vi "Simple H5Dwrite (Variant).vi"(0 "HDF5 Location Ref":T2, 1 "Close Dataset (T)":bool=TRUE, 2 "Compression Level (0-disabled)":i32 min=0 max=9 step=1, 3 "Chunk size":i32[](array[numeric]), 5 "Dataset Path":string, 9 "Unlimited  dataset (F)":bool, 11 "error in (no error)":errorcluster, 12 "operation (open or create)":T1=enum."open or create", 14 "Data":variant) -> (4 "HDF5 Location Ref out":T2, 6 "HDF5 Dataset Ref out":T2, 15 "error out":errorcluster)   [LabVIEW 2017]
doc: "Writes data into a dataset."
uses:
  <vilib>/UPVI/lvhdf5/library.llb/HDF5 Ref.ctl
  <vilib>/UPVI/lvhdf5/dataset.llb/LVH5D Operation.ctl
  <vilib>/UPVI/lvhdf5/common.llb/To HDF5 Ref.vi
panel:
  # "LVHDF5 Toolkit\nCopyright (c) 2005-2013 by Jason D. Sommerville\nCopyright (c) 2014 by UPVI, LLC.\n\nThis use and distribution of this file is governed by the terms found in \nLICENSE.txt distributed with this toolkit and installed at\n <user.lib>\\_lvhdf5\\LICENSE.txt"
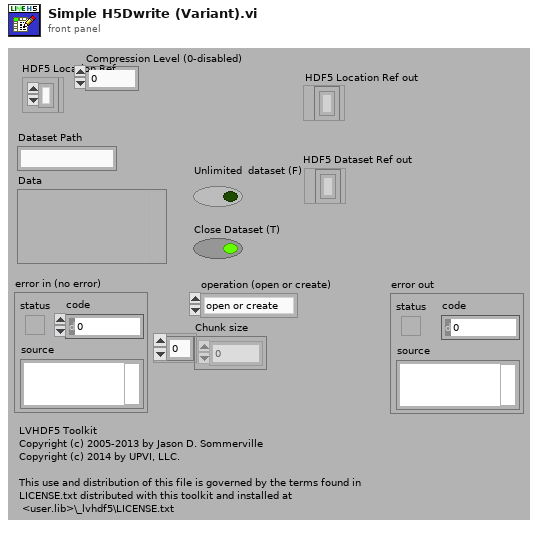
[diagram p1: front panel]
types:
  T1 = typedef "LVH5D Operation.ctl" = enum16{"open", "replace", "create", "open or create", "create or replace", "create or replace with confirmation"}
  T2 = typedef "HDF5 Ref.ctl" = refnum<k1>
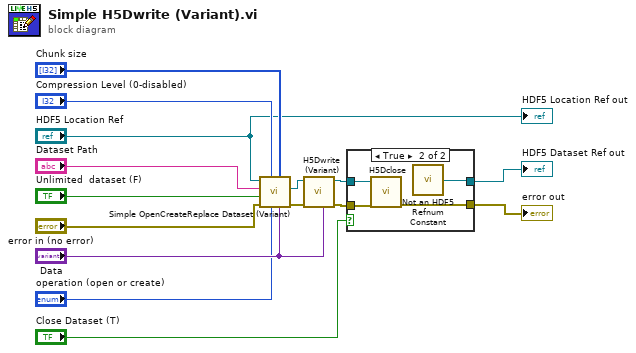
[diagram p0: block diagram]
diagram:
  n1 = call <vilib>:"Simple OpenCreateReplace Dataset (Variant).vi"("Datatype and Dataspace"="Data", "Chunk size"="Chunk size", "operation (open or create)"="operation (open or create)", "Compression Level (0-disabled)"="Compression Level (0-disabled)", "error in (no error)"="error in (no error)", "Unlimited  dataset (F)"="Unlimited  dataset (F)", "Dataset Path"="Dataset Path", "HDF5 Ref"="HDF5 Location Ref") -> ("error out"=w1:errorcluster, "HDF5 Dataset Ref out"=w2:T2)  [unwired: 1 in, 1 out]
  n2 = call <vilib>:"H5Dwrite (Variant).vi"("Data"="Data", "error in (no error)"=w1, "HDF5 Dataset Ref"=w2) -> ("error out"=w3:errorcluster, "HDF5 Ref out"=w4:T2)  [unwired: 7 in]
  n3 = case shown="True" "Close Dataset (T)" {
    tunnel: w4 -> [w17 w21]
    tunnel: [w16 w20] -> w9
    tunnel: w3 -> [w16 w19]
    tunnel: [w17 w18] -> w15
    frame False {
    }
    frame True {
      n4 = call <vilib>:"H5Dclose.vi"("error in (no error)"=w19, "HDF5 Dataset Ref"=w21) -> ("error out"=w20:errorcluster)  [unwired: 7 in]
      n5 = call <vilib>:"Not an HDF5 Refnum Constant.vi"() -> ("HDF5 Ref"=w18:T2)
    }
  }
  "error out" <- w9
  "HDF5 Dataset Ref out" <- w15
  "HDF5 Location Ref out" <- "HDF5 Location Ref"
